vi "testUnsignedChar.vi"() -> ()   [LabVIEW 2014]
uses:
  USBAnalyzerEllisysDll/Debug/USBAnalyzerEllisysDll.dll
panel:
  out "tabchar":u8[](array[numeric])
  out "size":i32
  out "return type 2":i32
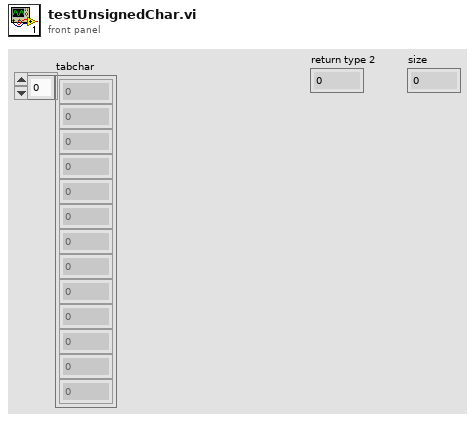
[diagram p1: front panel]
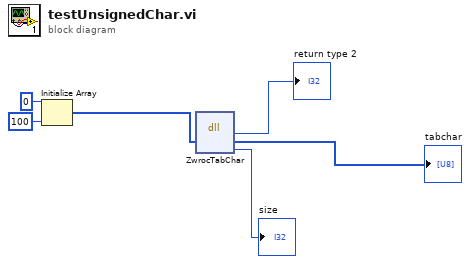
[diagram p0: block diagram]
diagram:
  n1 = Initialize Array(u8 0 ("element"), 100 ("dimension size")) -> (w1:u8[])
  n2 = dll-call lib="PTH2labs CUsersMichał\tDocumentsEllisysAnalyzerUSBAnalyzerEllisysDllDebugUSBAnalyzerEllisysDll.dll" fn="ZwrocTabChar"("tabchar"=w1) -> ("return type"=→"return type 2":i32, "tabchar"=→"tabchar":u8[], "size"=→"size":i32)  [unwired: 4 in, 2 out]
